vi "Autonomous Independent.vi"   [LabVIEW 2016]
doc: "This VI is called when autonomous begins, and will automatically be terminated when autonomous ends. You can carry out timed or sensor driven robot movement independently without needing to return to the caller."
uses:
  <vilib>/Rock Robotics/WPI/SafetyOutput/WPI_SafetyOutputConfigMenu.ctl
  <vilib>/Rock Robotics/WPI/Solenoid/WPI_SolenoidValue.ctl
  <vilib>/Rock Robotics/WPI/Utilities/WPI_GetSetVariantRefNum.vi
  <vilib>/Rock Robotics/Network Tables/NT Write Numeric Array.vi
  <vilib>/Rock Robotics/Network Tables/NT Read String.vi
  <vilib>/Rock Robotics/WPI/Solenoid/WPI_SolenoidSetEnum.vi
  <vilib>/Rock Robotics/WPI/RobotDrive/WPI_RobotDriveMecanumDrive_Cartesian.vi
panel:
  # "Be sure to right-click and choose Data Operations>>Make Current Value default if you want to save the array values with the VI"
types:
  T1 = typedef "WPI_JoystickDevRef.ctl" = cluster{"Device":T2}
  T2 = typedef "WPI_JoystickDeviceEnum.ctl" = enum16{"USB 0", "USB 1", "USB 2", "USB 3", "USB 4", "USB 5"}
  T3 = typedef "WPI_SafetyOutputConfigMenu.ctl" = enum16{"Enable", "Disable"}
  T4 = typedef "WPI_SolenoidValue.ctl" = enum16{"Off", "On", "Forward", "Reverse"}
  T5 = typedef "WPI_RobotDriveDevRef.ctl" = cluster{"DevStatus":errorcluster, "Motors[]":T6[], "Square Inputs":bool, "Max Output":dbl}
  T6 = typedef "WPI_MotorControlDeviceRef.ctl" = cluster{"DeviceStatus":errorcluster, "Type":T7, "PWM":cluster{"PWM Channel":T8, "DeadBand":T9}, "CAN":cluster{"Device Number":u8, "SetOutput VI Ref":variant, "GetOutput VI Ref":variant, "Enable VI Ref":variant, "Disable VI Ref":variant, "Data":variant}, "Invert":bool}
  T7 = typedef "WPI_MotorControlType.ctl" = enum16{"PWM", "CAN"}
  T8 = typedef "FPGA_DIOPWMChannel.ctl" = enum8{"PWM 0", "PWM 1", "PWM 2", "PWM 3", "PWM 4", "PWM 5", "PWM 6", "PWM 7", "PWM 8", "PWM 9", "PWM MXP 0", "PWM MXP 1", "PWM MXP 2", "PWM MXP 3", "PWM MXP 4", "PWM MXP 5", "PWM MXP 6", "PWM MXP 7", "PWM MXP 8", "PWM MXP 9", "Invalid"}
  T9 = typedef "WPI_PWMDeadband.ctl" = cluster{"Name":string, "maxPositivePwm":i32, "minPositivePwm":i32, "centerPwm":i32, "maxNegativePwm":i32, "minNegativePwm":i32, "angularRange":u16}
  T10 = typedef "WPI_SolenoidDevRef.ctl" = cluster{"DevStatus":errorcluster, "Pneumatics Control Module":u8, "Forward Solenoid Channel":T11, "Reverse Solenoid Channel":T11}
  T11 = typedef "WPI_SolenoidChannel.ctl" = enum8{"Solenoid 0", "Solenoid 1", "Solenoid 2", "Solenoid 3", "Solenoid 4", "Solenoid 5", "Solenoid 6", "Solenoid 7", "Invalid"}
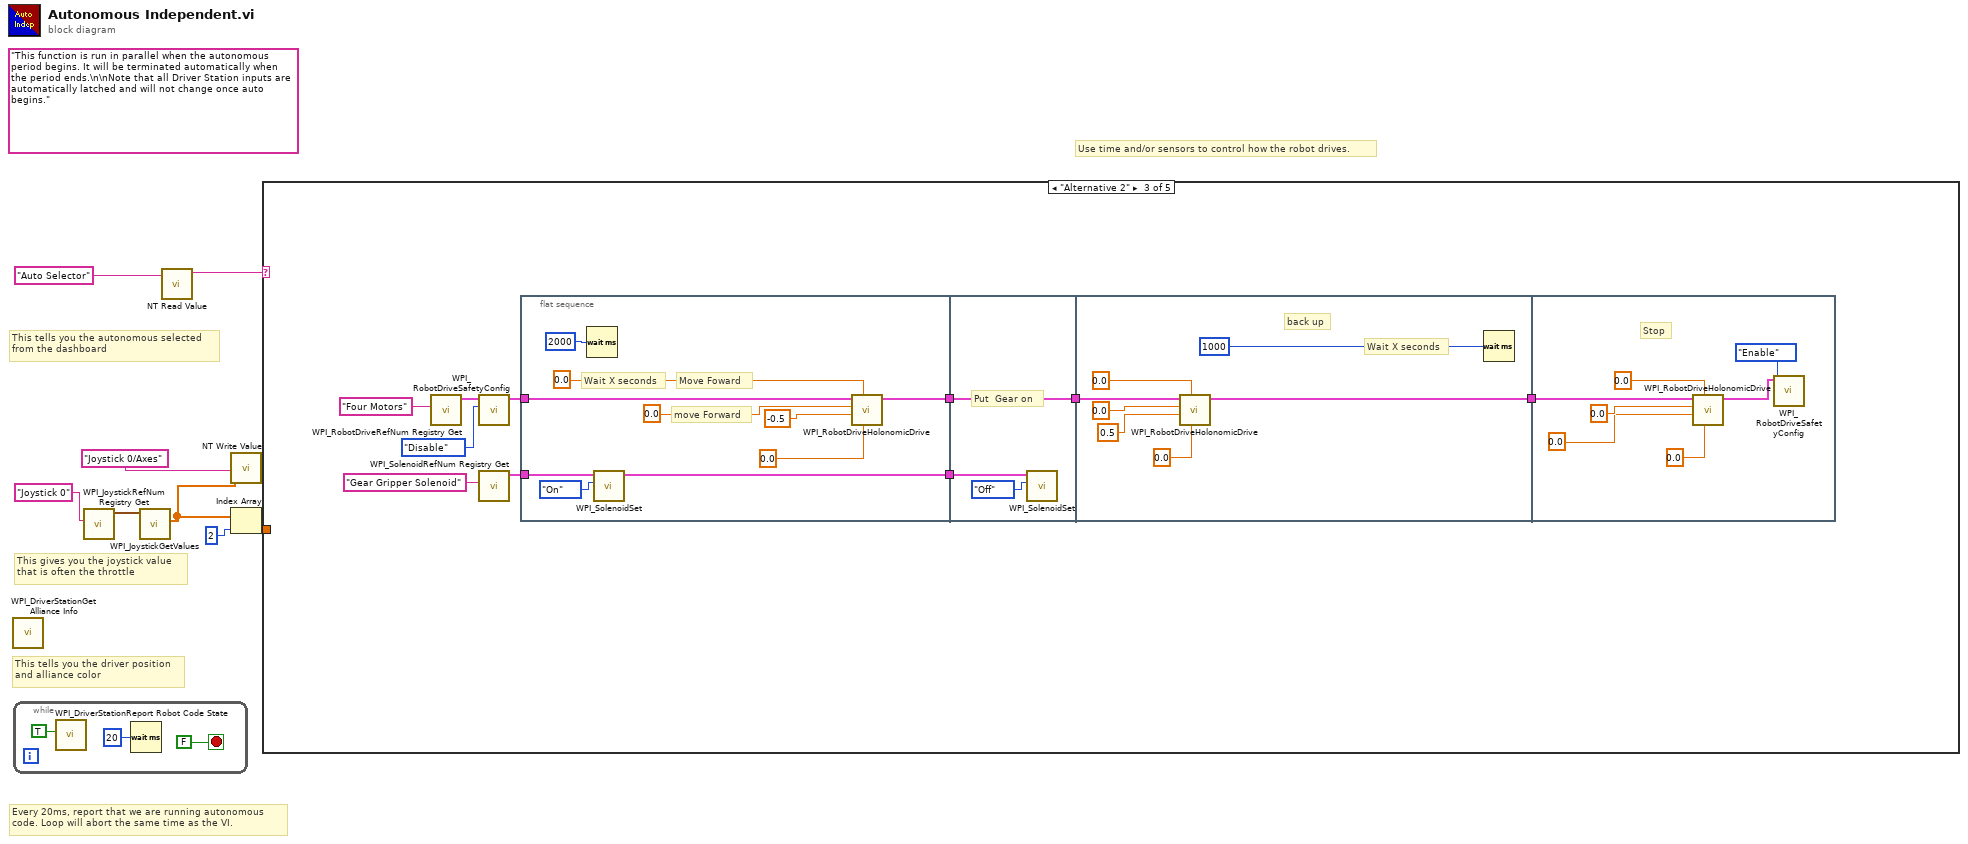
[diagram p0: block diagram]
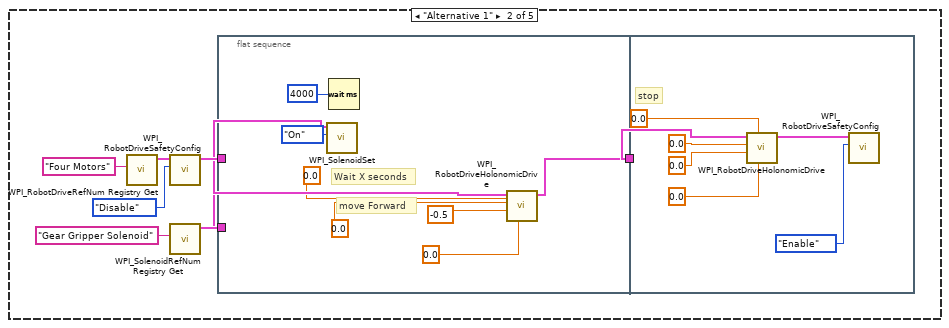
[diagram p3: hidden frame]
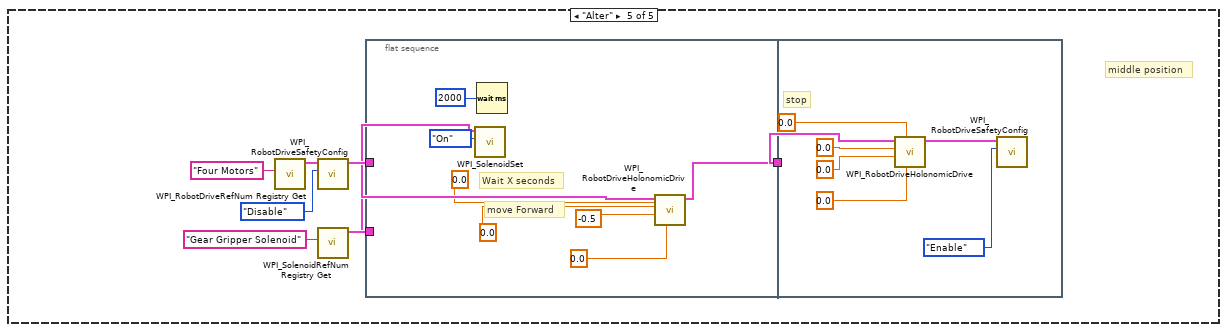
[diagram p5: hidden frame]
diagram:
  (unwired) "This function is run in parallel when the autonomous period begins. It will be terminated automatically when the period ends.\n\nNote that all Driver Station inputs are automatically latched and will not change once auto begins."
  # "This tells you the autonomous selected\nfrom the dashboard"
  # "Every 20ms, report that we are running autonomous\ncode. Loop will abort the same time as the VI."
  # "This gives you the joystick value\nthat is often the throttle"
  # "Use time and/or sensors to control how the robot drives."
  # "This tells you the driver position\nand alliance color"
  n1 = call <vilib>:"WPI_DriverStationGet Alliance Info.vi"() -> ()  [unwired: 12 out]
  n2 = while {
    stop <- FALSE stop-if-true
    n3 = call <vilib>:"WPI_DriverStationReport Robot Code State.vi"("Autonomous"=TRUE) -> ()  [unwired: 10 in, 1 out]
    n4 = Wait (ms)(milliseconds to wait=u32 20) -> ()  [unwired: 1 out]
  }
  n5 = call <vilib>:"WPI_JoystickRefNum Registry Get.vi"("refnum name"="Joystick 0") -> ("JoystickDevRef"=w7:T1)  [unwired: 1 in, 9 out]
  n6 = call <vilib>:"WPI_JoystickGetValues.vi"("JoystickDevRef"=w7) -> ("Axes"=w1:dbl[])  [unwired: 6 in, 4 out]
  n7 = call-poly <vilib>:"NT Read Value.vi"("Name"="Auto Selector") -> ("String"=w4:string)  [unwired: 9 in, 1 out]
  n8 = call-poly <vilib>:"NT Write Value.vi"("Numeric Array"=w1, "Name"="Joystick 0/Axes") -> ()  [unwired: 9 in, 1 out]
  n9 = Index Array(array=w1, index=u32 2 ("milliseconds to wait")) -> (element=w3:dbl)
  n10 = case shown="\"Alternative 2\"" w4 {
    tunnel: w3 -> [_ _ _ _ _]
    frame Default {
      # "You can put your main auto here, or you can right-click on the case and make any\nother frame be the default case."
      # "This is the frame that will execute if no selection is made, or if it is not recognized"
    }
    frame "Alternative 1" {
      n11 = call <vilib>:"WPI_RobotDriveRefNum Registry Get.vi"("refnum name"="Four Motors") -> ("RobotDriveDevRef"=w16:T5)  [unwired: 9 in, 1 out]
      n12 = call <vilib>:"WPI_RobotDriveSafetyConfig.vi"("mode"=WPI_SafetyOutputConfigMenu."Disable", "RobotDriveDevRef"=w16) -> ("RobotDriveDevRef"=w15:T5)  [unwired: 8 in, 1 out]
      n13 = call <vilib>:"WPI_SolenoidRefNum Registry Get.vi"("refnum name"="Gear Gripper Solenoid") -> ("SolenoidDevRef"=w13:T10)  [unwired: 9 in, 1 out]
      n14 = flat-sequence {
        tunnel: w15 -> [w27]
        tunnel: [w26] -> w18
        tunnel: w13 -> [w20]
        tunnel: w18 -> [w34]
        frame #0 {
          # "Wait X seconds"
          # "move Forward"
          n15 = call-poly <vilib>:"WPI_SolenoidSet.vi"("Value"=WPI_SolenoidValue."On", "SolenoidDevRef"=w20) -> ()  [unwired: 8 in, 2 out]
          n16 = Wait (ms)(milliseconds to wait=u32 4000) -> ()  [unwired: 1 out]
          n17 = call-poly <vilib>:"WPI_RobotDriveHolonomicDrive.vi"("Rotation"=0.0, "Gyro Angle"=0.0, "Y"=-0.5, "X"=0.0, "RobotDriveDevRef"=w27) -> ("RobotDriveDevRef"=w26:T5)  [unwired: 4 in, 2 out]
        }
        frame #1 {
          # "stop"
          n18 = call-poly <vilib>:"WPI_RobotDriveHolonomicDrive.vi"("Rotation"=0.0, "Gyro Angle"=0.0, "Y"=0.0, "X"=0.0, "RobotDriveDevRef"=w34) -> ("RobotDriveDevRef"=w29:T5)  [unwired: 4 in, 2 out]
          n19 = call <vilib>:"WPI_RobotDriveSafetyConfig.vi"("mode"=WPI_SafetyOutputConfigMenu."Enable", "RobotDriveDevRef"=w29) -> ()  [unwired: 8 in, 2 out]
        }
      }
    }
    frame "Alternative 2" {
      n20 = call <vilib>:"WPI_RobotDriveRefNum Registry Get.vi"("refnum name"="Four Motors") -> ("RobotDriveDevRef"=w42:T5)  [unwired: 9 in, 1 out]
      n21 = call <vilib>:"WPI_RobotDriveSafetyConfig.vi"("mode"=WPI_SafetyOutputConfigMenu."Disable", "RobotDriveDevRef"=w42) -> ("RobotDriveDevRef"=w41:T5)  [unwired: 8 in, 1 out]
      n22 = call <vilib>:"WPI_SolenoidRefNum Registry Get.vi"("refnum name"="Gear Gripper Solenoid") -> ("SolenoidDevRef"=w39:T10)  [unwired: 9 in, 1 out]
      n23 = flat-sequence {
        tunnel: w41 -> [w54]
        tunnel: [w53] -> w44
        tunnel: w39 -> [w47]
        tunnel: [w45] -> w37
        tunnel: w44 -> [w55]
        tunnel: w37 -> [w57]
        tunnel: [w55] -> w36
        tunnel: w36 -> [w60]
        tunnel: [w59] -> w35
        tunnel: w35 -> [w68]
        frame #0 {
          # "Move Foward"
          # "Wait X seconds"
          # "move Forward"
          n24 = Wait (ms)(milliseconds to wait=u32 2000) -> ()  [unwired: 1 out]
          n25 = call-poly <vilib>:"WPI_SolenoidSet.vi"("Value"=WPI_SolenoidValue."On", "SolenoidDevRef"=w47) -> ("SolenoidDevRef"=w45:T10)  [unwired: 8 in, 1 out]
          n26 = call-poly <vilib>:"WPI_RobotDriveHolonomicDrive.vi"("Rotation"=0.0, "Gyro Angle"=0.0, "Y"=-0.5, "X"=0.0, "RobotDriveDevRef"=w54) -> ("RobotDriveDevRef"=w53:T5)  [unwired: 4 in, 2 out]
        }
        frame #1 {
          # "Put  Gear on"
          n27 = call-poly <vilib>:"WPI_SolenoidSet.vi"("Value"=WPI_SolenoidValue."Off", "SolenoidDevRef"=w57) -> ()  [unwired: 8 in, 2 out]
        }
        frame #2 {
          # "Wait X seconds"
          # "back up"
          n28 = call-poly <vilib>:"WPI_RobotDriveHolonomicDrive.vi"("Rotation"=0.0, "Gyro Angle"=0.0, "Y"=0.5, "X"=0.0, "RobotDriveDevRef"=w60) -> ("RobotDriveDevRef"=w59:T5)  [unwired: 4 in, 2 out]
          n29 = Wait (ms)(milliseconds to wait=u32 1000) -> ()  [unwired: 1 out]
        }
        frame #3 {
          # "Stop"
          n30 = call-poly <vilib>:"WPI_RobotDriveHolonomicDrive.vi"("Rotation"=0.0, "Gyro Angle"=0.0, "Y"=0.0, "X"=0.0, "RobotDriveDevRef"=w68) -> ("RobotDriveDevRef"=w65:T5)  [unwired: 4 in, 2 out]
          n31 = call <vilib>:"WPI_RobotDriveSafetyConfig.vi"("mode"=WPI_SafetyOutputConfigMenu."Enable", "RobotDriveDevRef"=w65) -> ()  [unwired: 8 in, 2 out]
        }
      }
    }
    frame "Your Turn" {
    }
    frame "Alter" {
      # "middle position"
      n32 = call <vilib>:"WPI_RobotDriveRefNum Registry Get.vi"("refnum name"="Four Motors") -> ("RobotDriveDevRef"=w76:T5)  [unwired: 9 in, 1 out]
      n33 = call <vilib>:"WPI_RobotDriveSafetyConfig.vi"("mode"=WPI_SafetyOutputConfigMenu."Disable", "RobotDriveDevRef"=w76) -> ("RobotDriveDevRef"=w75:T5)  [unwired: 8 in, 1 out]
      n34 = call <vilib>:"WPI_SolenoidRefNum Registry Get.vi"("refnum name"="Gear Gripper Solenoid") -> ("SolenoidDevRef"=w73:T10)  [unwired: 9 in, 1 out]
      n35 = flat-sequence {
        tunnel: w75 -> [w87]
        tunnel: [w86] -> w78
        tunnel: w73 -> [w80]
        tunnel: w78 -> [w94]
        frame #0 {
          # "Wait X seconds"
          # "move Forward"
          n36 = call-poly <vilib>:"WPI_SolenoidSet.vi"("Value"=WPI_SolenoidValue."On", "SolenoidDevRef"=w80) -> ()  [unwired: 8 in, 2 out]
          n37 = Wait (ms)(milliseconds to wait=u32 2000) -> ()  [unwired: 1 out]
          n38 = call-poly <vilib>:"WPI_RobotDriveHolonomicDrive.vi"("Rotation"=0.0, "Gyro Angle"=0.0, "Y"=-0.5, "X"=0.0, "RobotDriveDevRef"=w87) -> ("RobotDriveDevRef"=w86:T5)  [unwired: 4 in, 2 out]
        }
        frame #1 {
          # "stop"
          n39 = call-poly <vilib>:"WPI_RobotDriveHolonomicDrive.vi"("Rotation"=0.0, "Gyro Angle"=0.0, "Y"=0.0, "X"=0.0, "RobotDriveDevRef"=w94) -> ("RobotDriveDevRef"=w89:T5)  [unwired: 4 in, 2 out]
          n40 = call <vilib>:"WPI_RobotDriveSafetyConfig.vi"("mode"=WPI_SafetyOutputConfigMenu."Enable", "RobotDriveDevRef"=w89) -> ()  [unwired: 8 in, 2 out]
        }
      }
    }
  }
